vi "Nested Exist.vi"(11 "Ex Queue Actor in":refnum<class "Ex Queue Actor.lvclass">) -> (2 "Nested Exist?":bool)   [LabVIEW 2021, in "Ex Queue Actor.lvlib" / "Ex Queue Actor.lvclass"]
uses:
  Ex Queue Actor.lvclass
  Ex Queue Actor.lvclass/Ex Queue Actor.ctl
  Actor/Queue Actor/Queue Actor.lvclass
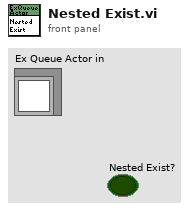
[diagram p1: front panel]
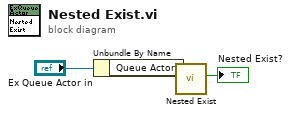
[diagram p0: block diagram]
diagram:
  n1 = Unbundle By Name("Ex Queue Actor in") -> ("Queue Actor"=w2:refnum<class "Queue Actor.lvclass">)
  n2 = call-dynamic "Nested Exist.vi"("Queue Actor in"=w2) -> ("Nested Exist?"=→"Nested Exist?":bool)  [unwired: 10 in]
